vi "Compress Images.vi"(7 "Front Panel in":T1, 11 "Frame Data":T2(array[cluster])) -> (3 "Images":cluster{"Image":T1, "Child Indexes":i32[]}[](array[cluster]))   [LabVIEW 2026]
doc: "This vi takes an array of image datas, and converts each of them into a Base64 compression string. It then returns an array with information for each image, including the rectangle, compressed string, the relative time it will appear for in a SVG, and the indexes for both the frame's owner and children. An array of the uncompressed image datas are also returned."
uses:
  <vilib>/picture/picture.llb/imagedata.ctl
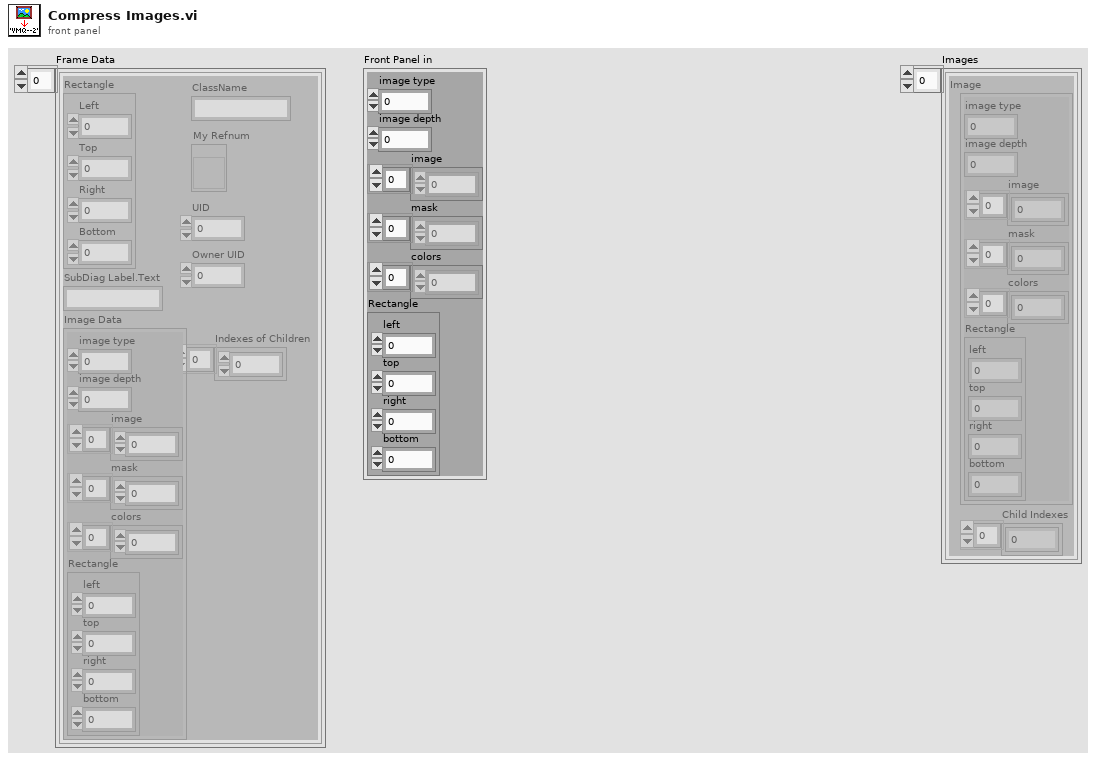
[diagram p1: front panel]
types:
  T1 = typedef "imagedata.ctl" = cluster{"image type":i32, "image depth":i32, "image":u8[], "mask":u8[], "colors":u32[], "Rectangle":cluster{"left":i16, "top":i16, "right":i16, "bottom":i16}}
  T2 = cluster{"Rectangle":cluster{"Left":i32, "Top":i32, "Right":u32, "Bottom":u32}, "SubDiag Label.Text":string, "Image Data":T1, "ClassName":string, "My Refnum":refnum<vi>, "UID":i32, "Owner UID":i32, "Indexes of Children":i32[]}[]
  T3 = cluster{"Front Panel":T1, "Child Indexes":i32[]}[]
  T4 = cluster{"Front Panel in":T1, "Child Indexes in":i32[]}
  T5 = cluster{"Rectangle":cluster{"Left":i32, "Top":i32, "Right":u32, "Bottom":u32}, "Image Data":T1, i32, "Indexes of Children":i32[]}
  T6 = cluster{"Left":i32, "Top":i32, "Right":u32, "Bottom":u32}
  T7 = cluster{"Rectangle":cluster{"Left":i32, "Top":i32, "Right":u32, "Bottom":u32}, "Image Data":T1, i32, i32[]}
  T8 = cluster{"Image Data":T1, "Indexes of Children":i32[]}
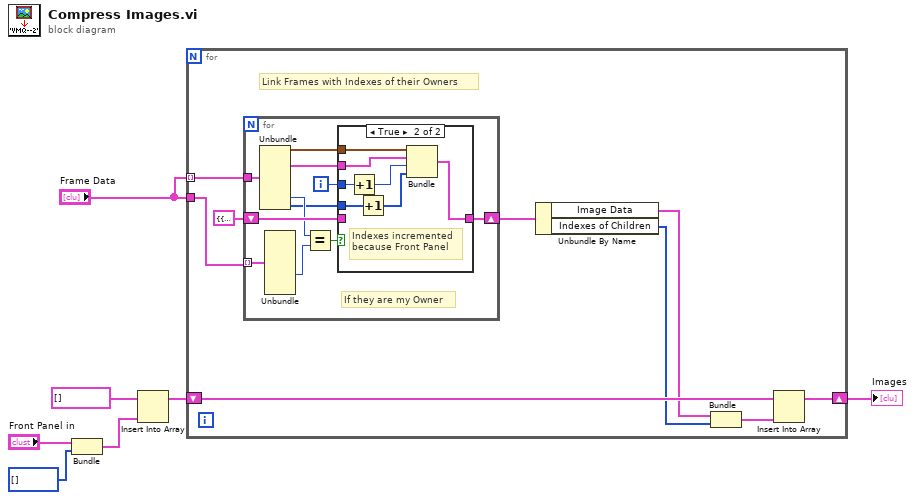
[diagram p0: block diagram]
diagram:
  n1 = Bundle("Front Panel in"="Front Panel in", "Child Indexes in"=i32[] []) -> (w5:T4)  [unwired: 1 in]
  n2 = Insert Into Array(array=T3 [], new element=w5) -> (w1:T3)  [unwired: 1 in]
  n3 = for {
    tunnel: "Frame Data" -> [w16] mode=indexing
    tunnel: "Frame Data" -> [w15]
    shift-right: [w13] -> w4
    shift-left: w1 -> [w14]
    # "Link Frames with Indexes of their Owners"
    n4 = for {
      tunnel: w15 -> [w26] mode=indexing
      tunnel: w16 -> [w27]
      shift-right: [w21] -> w10
      shift-left: T5 {"Rectangle"={"Left"=0, "Top"=0, "Right"=0, "Bottom"=0}, "Image Data"={"image type"=0, "image depth"=0, "image"=[], "mask"=[], "colors"=[], "Rectangle"={"left"=0, "top"=0, "right"=0, "bottom"=0}}, 0, "Indexes of Children"=[]} -> [w22]
      i -> [w18]
      # "If they are my Owner"
      n5 = Unbundle(w27) -> ("Rectangle"=w24:T6, "Image Data"=w23:T1, "Owner UID"=w20:i32, "Indexes of Children"=w17:i32[])  [unwired: 4 out]
      n6 = Unbundle(w26) -> ("UID"=w19:i32)  [unwired: 7 out]
      n7 = Equal?(x=w20, y=w19) -> (x = y?=w25:bool)
      n8 = case shown="True" w25 {
        tunnel: w24 -> [_ w35]
        tunnel: w23 -> [_ w34]
        tunnel: [w28 w33] -> w21
        tunnel: w22 -> [w28 _]
        tunnel: w18 -> [_ w32]
        tunnel: w17 -> [_ w30]
        frame False {
        }
        frame True {
          # "Indexes incremented\nbecause Front Panel"
          n9 = Increment(x=w32) -> (x+1=w31:i32)
          n10 = Increment(x=w30) -> (x+1=w29:i32[])
          n11 = Bundle("Rectangle"=w35, "Image Data"=w34, w31, w29) -> (w33:T7)  [unwired: 1 in]
        }
      }
    }
    n12 = Unbundle By Name(w10) -> ("Image Data"=w9:T1, "Indexes of Children"=w8:i32[])
    n13 = Bundle("Image Data"=w9, "Indexes of Children"=w8) -> (w11:T8)  [unwired: 1 in]
    n14 = Insert Into Array(array=w14, new element=w11) -> (w13:T3)  [unwired: 1 in]
  }
  "Images" <- w4
